vi "Feed.vi"() -> ()   [LabVIEW 2014]
uses:
  subVI/version.vi
panel:
  in  "닫기":bool
  in  "전송":bool
  in  "Message":string caption="메시지"
  # "개발자에게 피드백"
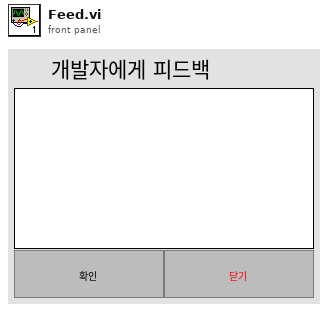
[diagram p1: front panel]
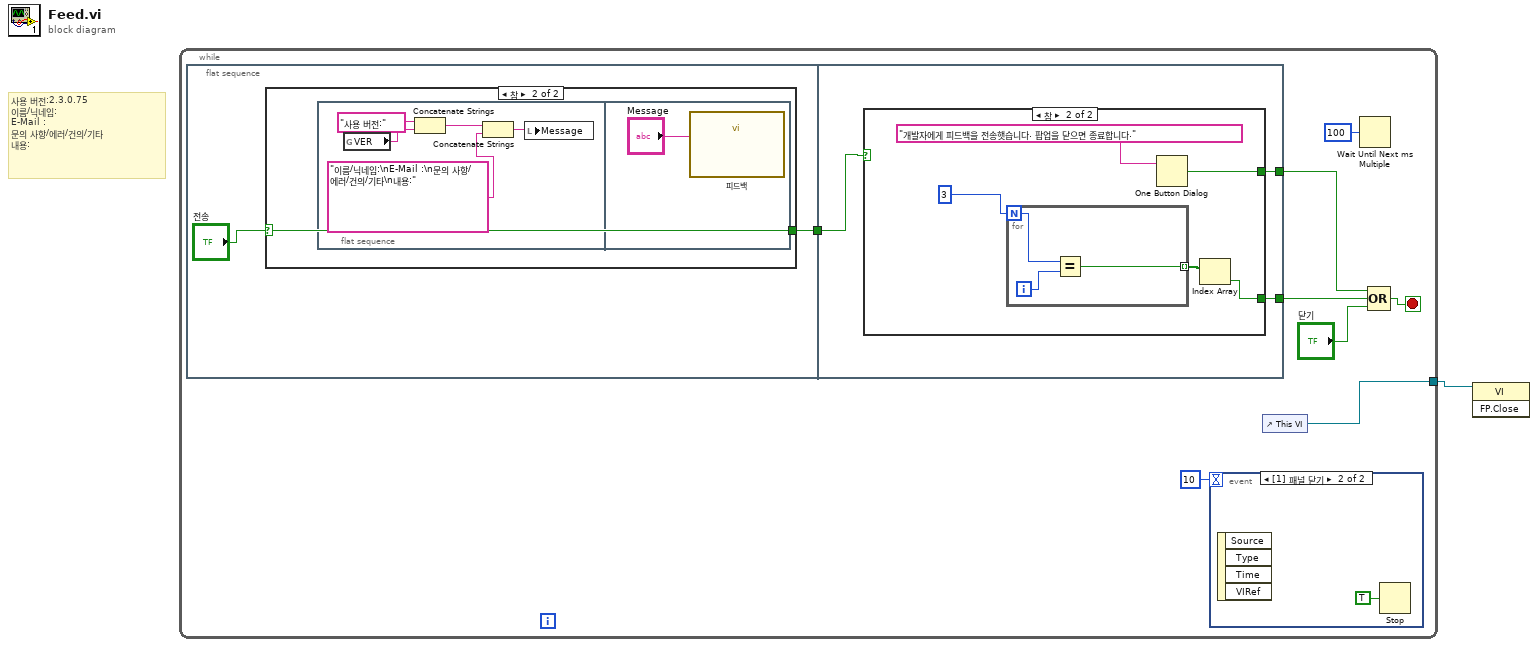
[diagram p0: block diagram]
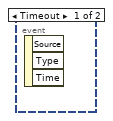
[diagram p2: hidden frame]
diagram:
  # "사용 버전:2.3.0.75\n이름/닉네임:\nE-Mail :\n문의 사항/에러/건의/기타\n내용:"
  n1 = while {
    tunnel: [w9] -> w1
    stop <- w4 stop-if-true
    n2 = flat-sequence {
      tunnel: [w11] -> w8
      tunnel: w8 -> [w22]
      tunnel: [w21] -> w5
      tunnel: [w20] -> w6
      frame #0 {
        n3 = case shown="참" "전송" {
          selector: "전송" -> [_ w13]
          tunnel: [_ w13] -> w11
          frame False {
          }
          frame True {
            n4 = flat-sequence {
              frame #0 {
                n5 = global read "version.vi" "VER"() -> (w14:string)
                n6 = Concatenate Strings("사용 버전:" ("문자열"), w14) -> (w16:string)
                n7 = Concatenate Strings(w16, "이름/닉네임:\nE-Mail :\n문의 사항/에러/건의/기타\n내용:" ("문자열")) -> (w18:string)
                n8 = local write "Message"(w18) -> ()
              }
              frame #1 {
                n9 = call "피드백"("Message"="Message") -> ()  [unwired: 10 in, 1 out]
              }
            }
          }
        }
      }
      frame #1 {
        n10 = case shown="참" w22 {
          tunnel: [_ w26] -> w21
          tunnel: [_ w23] -> w20
          frame False {
          }
          frame True {
            n11 = for {
              N: 3 -> [w29]
              tunnel: [w28] -> w24 mode=indexing
              i -> [w30]
              n12 = Equal?(x=w29, y=w30) -> (x = y?=w28:bool)
            }
            n13 = One Button Dialog(message="개발자에게 피드백을 전송햇습니다. 팝업을 닫으면 종료합니다." ("메시지")) -> (true=w26:bool)  [unwired: 1 in]
            n14 = Index Array(array=w24) -> (element=w23:bool)  [unwired: 1 in]
          }
        }
      }
    }
    n15 = event shown="[1] 패널 닫기" {
      selector: _ -> [_ _]
      dyn-events: _ -> [_ _]
      timeout: 10 -> [_ _]
      event Timeout {
        n16 = event-data() -> ()  [unwired: 1 in, 3 out]
      }
      event Panel Close {
        n17 = event-data() -> ()  [unwired: 1 in, 4 out]
        n18 = Stop(stop? (T)=TRUE ("정지? (참)")) -> ()
      }
    }
    n19 = control-ref of="This VI"() -> (w9:refnum<vi>)
    n20 = Wait Until Next ms Multiple(millisecond multiple=u32 100 ("ms 배수")) -> ()  [unwired: 1 out]
    n21 = Compound Arithmetic op=OR(w5, w6, "닫기") -> (w4:bool)
  }
  n22 = invoke class="VI" method="FP.Close"(reference=w1) -> ()  [unwired: 2 in, 3 out]
